vi "Strain Props.vi"(8 "error in (no error)":errorcluster, 11 "Board Info for checking":T1) -> (0 "error out":errorcluster, 2 "scaling info out":variant, 3 "bridge info out":variant)   [LabVIEW 2010, in "PXIe-433x Custom Device.lvlib"]
uses:
  PXIe-433x Custom Device.lvlib
  Strain Bridge Information.ctl
  Strain Information.ctl
  Min Value.ctl
  Max Value.ctl
  Board Info for checking settings.ctl
  Sensor Type.ctl
panel:
  out "Tab Control":enum32{"No Error", "No Check", "Error"}(tab)
  out "Valid":bool=TRUE
  out "No Check":bool=TRUE
  in  "No Error Check Details":bool
  in  "Error Details":bool
  out "Error Description":string
  out "Valid Configuration?":bool
  in  "stop":bool
  in  "Maximum Value":T2=0.05 caption="Strain"
  in  "Minimum Value":T3=-0.05 caption="Strain"
  in  "strain gage information":T4={"gage factor"=2.0, "nominal gage resistance"=350.0, "poisson ratio"=0.3} {"nominal gage resistance" format="%0.2f"; "poisson ratio" format="%0.2f"; "gage factor" format="%0.2f"}
  in  "bridge information":T5={"strain configuration"=10183, "lead wire resistance"=0.0, "initial bridge voltage"=0.0, "voltage excitation source"=10200, "voltage excitation value"=2.5} {"initial bridge voltage" format="%0.2f"; "voltage excitation source" items=["Internal"=10200, "External"=10167, "None"=10230]; "voltage excitation value" format="%0.2f"; "lead wire resistance" format="%0.2f"; "strain configuration" items=["Full Bridge I"=10183, "Full Bridge II"=10184, "Full Bridge III"=10185, "Half Bridge I"=10188, "Half Bridge II"=10189, "Quarter Bridge I"=10271, "Quarter Bridge II"=10272]}
  # "No Error"
  # "No Error Check"
  # "Error!"
  # "Ohm"
  # "V"
  # "V"
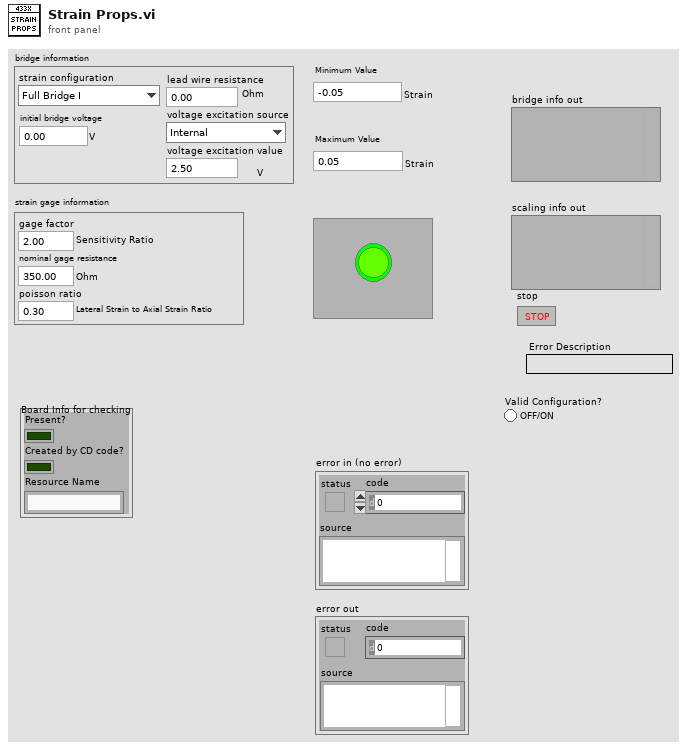
[diagram p1: front panel]
types:
  T1 = typedef "PXIe-433x Custom Device.lvlib/Board Info for checking settings.ctl" = cluster{"Present?":bool, "Created by CD code?":bool, "Resource Name":string}
  T2 = typedef "PXIe-433x Custom Device.lvlib/Max Value.ctl" = dbl
  T3 = typedef "PXIe-433x Custom Device.lvlib/Min Value.ctl" = dbl
  T4 = typedef "PXIe-433x Custom Device.lvlib/Strain Information.ctl" = cluster{"gage factor":dbl, "nominal gage resistance":dbl, "poisson ratio":dbl}
  T5 = typedef "PXIe-433x Custom Device.lvlib/Strain Bridge Information.ctl" = cluster{"strain configuration":i32, "lead wire resistance":dbl, "initial bridge voltage":dbl, "voltage excitation source":i32, "voltage excitation value":dbl}
  T6 = typedef "PXIe-433x Custom Device.lvlib/Sensor Type.ctl" = enum16{"Strain", "Force", "Pressure", "Torque"}
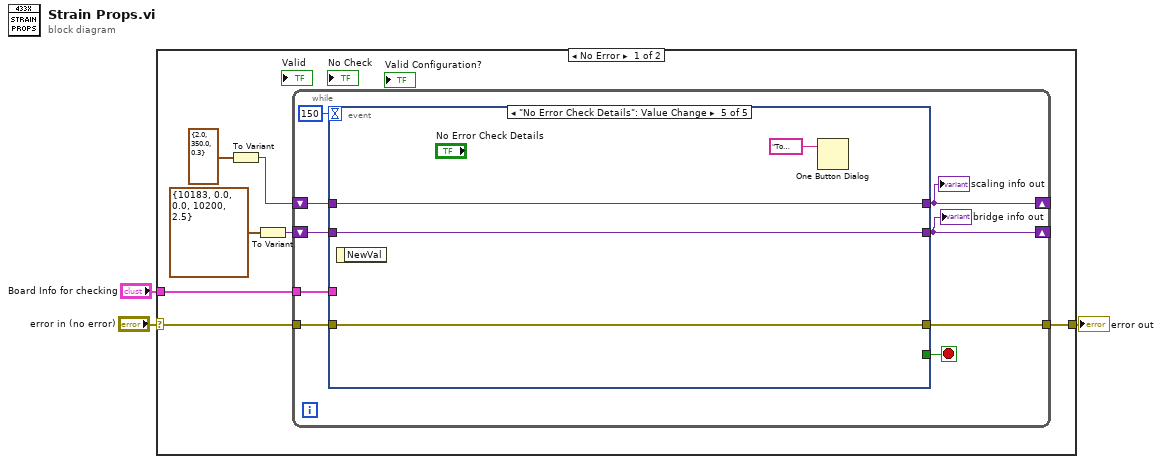
[diagram p0: block diagram]
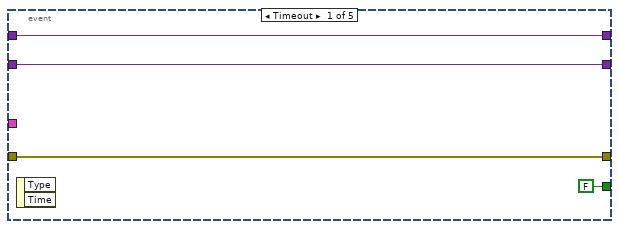
[diagram p2: hidden frame]
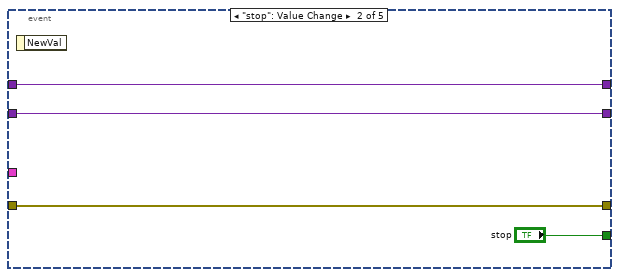
[diagram p3: hidden frame]
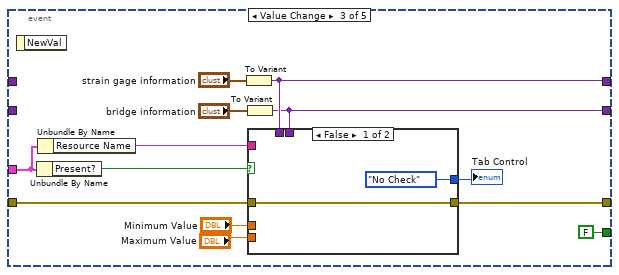
[diagram p4: hidden frame]
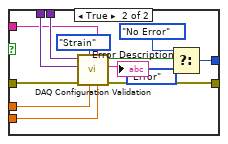
[diagram p5: hidden frame]
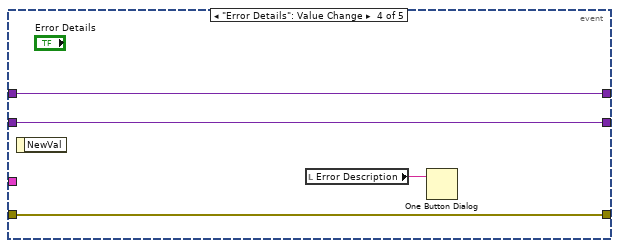
[diagram p6: hidden frame]
diagram:
  n1 = case shown="No Error" "error in (no error)" {
    selector: "error in (no error)" -> [w5 w64]
    tunnel: [w10 w64] -> w3
    tunnel: "Board Info for checking" -> [w4 _]
    frame No Error {
      n2 = To Variant(anything=T4 {"gage factor"=2.0, "nominal gage resistance"=350.0, "poisson ratio"=0.3} ("strain gage information")) -> (Variant=w6:variant)
      n3 = To Variant(anything=T5 {"strain configuration"=10183, "lead wire resistance"=0.0, "initial bridge voltage"=0.0, "voltage excitation source"=10200, "voltage excitation value"=2.5} ("bridge information")) -> (Variant=w9:variant)
      n4 = while {
        tunnel: w5 -> [w19]
        tunnel: [w17] -> w10
        shift-right: [w15] -> _
        shift-left: w6 -> [w14]
        shift-right: [w12] -> _
        shift-left: w9 -> [w13]
        tunnel: w4 -> [w11]
        stop <- w18 stop-if-true
        n5 = event shown="[4] \"No Error Check Details\": Value Change" {
          selector: _ -> [_ _ _ _ _]
          dyn-events: _ -> [_ _ _ _ _]
          timeout: 150 -> [_ _ _ _ _]
          tunnel: w19 -> [w22 w26 w39 w59 w63]
          tunnel: [FALSE ("stop") "stop" FALSE ("stop") _ _] -> w18
          tunnel: [w22 w26 w32 w59 w63] -> w17
          tunnel: [w21 w25 w31 w56 w61] -> w15
          tunnel: w14 -> [w21 w25 _ w56 w61]
          tunnel: [w20 w24 w30 w57 w62] -> w12
          tunnel: w13 -> [w20 w24 _ w57 w62]
          tunnel: w11 -> [_ _ w29 _ _]
          event Timeout {
            n6 = event-data() -> ()  [unwired: 1 in, 2 out]
          }
          event "stop": Value Change {
            n7 = event-data() -> ()  [unwired: 1 in, 1 out]
          }
          event Value Change {
            n8 = event-data() -> ()  [unwired: 1 in, 1 out]
            n9 = Unbundle By Name(w29) -> ("Present?"=w40:bool)
            n10 = Unbundle By Name(w29) -> ("Resource Name"=w28:string)
            n11 = To Variant(anything="strain gage information") -> (Variant=w31:variant)
            n12 = To Variant(anything="bridge information") -> (Variant=w30:variant)
            n13 = case shown="False" w40 {
              tunnel: w39 -> [w42 w55]
              tunnel: [w42 w48] -> w32
              tunnel: "Minimum Value" -> [_ w53]
              tunnel: "Maximum Value" -> [_ w52]
              tunnel: w31 -> [_ w50]
              tunnel: w30 -> [_ w51]
              tunnel: [enum32{"No Error", "No Check", "Error"}."No Check" ("Tab Control") w46] -> w33
              tunnel: w28 -> [_ w43]
              frame False {
              }
              frame True {
                n14 = call "DAQ Configuration Validation.vi"("Maximum Value"=w52, "DAQ Resource Name"=w43, "Minimum Value"=w53, "Sensor Type"=Sensor_Type."Strain", "error in"=w55, "scaling info"=w50, "bridge info"=w51) -> ("error IO"=w48:errorcluster, "Error Source"=→"Error Description":string, "Valid configuration?"=w44:bool)  [unwired: 2 in]
                n15 = Select(t=enum32{"No Error", "No Check", "Error"}."No Error" ("Tab Control"), s=w44, f=enum32{"No Error", "No Check", "Error"}."Error" ("Tab Control")) -> (s? t:f=w46:enum32{"No Error", "No Check", "Error"})
              }
            }
            "Tab Control" <- w33
          }
          event "Error Details": Value Change {
            n16 = event-data() -> ()  [unwired: 1 in, 1 out]
            n17 = local read "Error Description"() -> (w58:string)
            n18 = One Button Dialog(message=w58) -> ()  [unwired: 1 in, 1 out]
          }
          event "No Error Check Details": Value Change {
            n19 = event-data() -> ()  [unwired: 1 in, 1 out]
            n20 = One Button Dialog(message="To perform error checking during Edition time, code needs either a physical local PXIe-433x or simulated one. One simulated couldn't be created, no error checking will be performed while editing settings. Error checking will still be performed while deploying Custom-Device.") -> ()  [unwired: 1 in, 1 out]
          }
        }
        "scaling info out" <- w15
        "bridge info out" <- w12
      }
    }
    frame Error {
    }
  }
  "error out" <- w3
